vi "CreatemodulePicString.vi"(8 "Error In":errorcluster, 10 "input string":string, 11 "Slot Nr":i32) -> (0 "Error Out":errorcluster, 3 "Pic String Out":string)   [LabVIEW 2011]
uses:
  Controls/ModulePicCluster.ctl
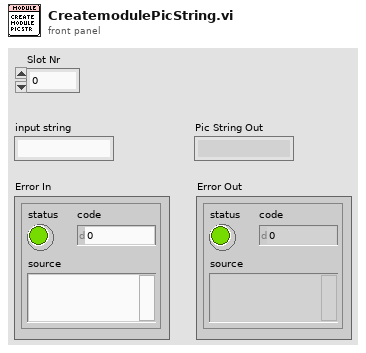
[diagram p1: front panel]
types:
  T1 = typedef "ModulePicCluster.ctl" = cluster{"Slot Nr":i32, "ModulePic":picture}
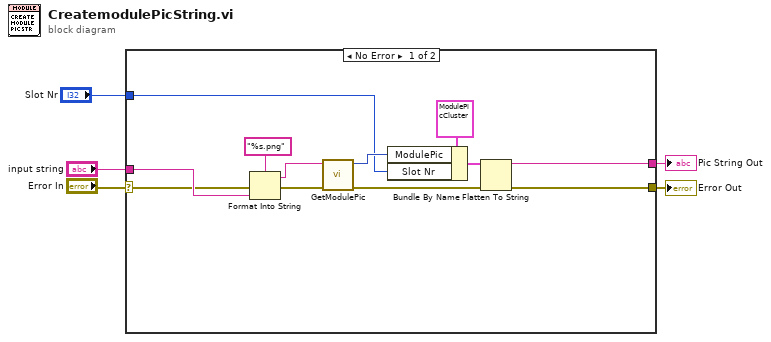
[diagram p0: block diagram]
diagram:
  n1 = case shown="No Error" "Error In" {
    selector: "Error In" -> [w14 w18]
    tunnel: "input string" -> [w15 _]
    tunnel: [w17 w18] -> w4
    tunnel: [w16 _] -> w2
    tunnel: "Slot Nr" -> [w7 _]
    frame No Error {
      n2 = Format Into String(format string="%s.png", error in=w14, w15) -> (resulting string=w10:string, error out=w8:errorcluster)  [unwired: 1 in]
      n3 = call "GetModulePic.vi"("Error In"=w8, "name"=w10) -> ("Error Out"=w6:errorcluster, "new picture"=w9:picture)  [unwired: 8 in]
      n4 = Bundle By Name(cluster=T1 {"Slot Nr"=0, "ModulePic"=bytes[0]}, "ModulePic"=w9, "Slot Nr"=w7) -> (w12:T1)
      n5 = Flatten To String(anything=w12, error in (no error)=w6) -> (data string=w16:string, error out=w17:errorcluster)  [unwired: 2 in, 1 out]
    }
    frame Error {
    }
  }
  "Error Out" <- w4
  "Pic String Out" <- w2
